vi "Add Copied Standalone VIs to Library.vi"(0 "project reference in":refnum<vi>, 5 "copied standalone VIs":cluster{"Lib path":path, "VI path":path}[](array[cluster]), 11 "error in":errorcluster) -> (4 "project reference out":refnum<vi>, 15 "error out":errorcluster)   [LabVIEW 2021, in "Multiple Converter.lvlib"]
uses:
  Multiple Converter.lvlib
  Converter Reusables/Converter Reusables.lvlib
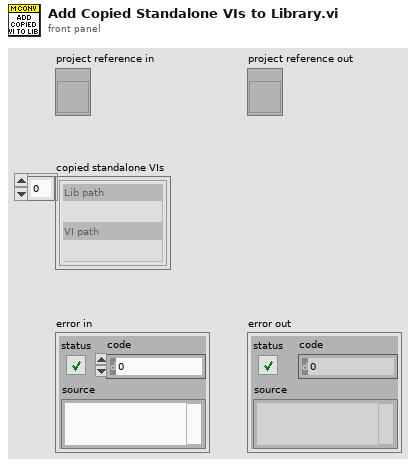
[diagram p1: front panel]
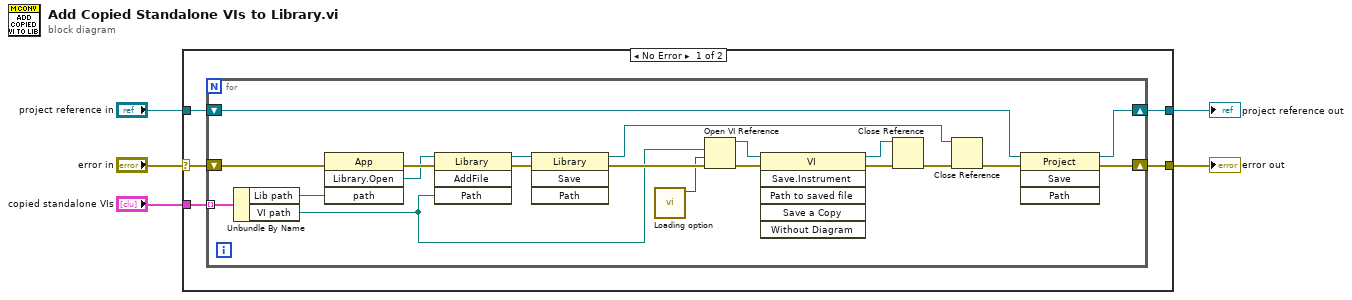
[diagram p0: block diagram]
diagram:
  n1 = case shown="No Error" "error in" {
    selector: "error in" -> [w10 w32]
    tunnel: [w9 w32] -> w4
    tunnel: "project reference in" -> [w8 w31]
    tunnel: [w7 w31] -> w2
    tunnel: "copied standalone VIs" -> [w6 _]
    frame No Error {
      n2 = for {
        shift-right: [w16] -> w9
        shift-left: w10 -> [w30]
        shift-right: [w14] -> w7
        shift-left: w8 -> [w15]
        tunnel: w6 -> [w11] mode=indexing
        n3 = Unbundle By Name(w11) -> ("Lib path"=w25:path, "VI path"=w22:path)
        n4 = invoke class="App" method="Library.Open"(error in=w30, "path"=w25) -> (error out=w29:errorcluster, "Open Library"=w24:refnum<vi>)  [unwired: 2 in, 2 out]
        n5 = invoke class="Library" method="AddFile"(reference=w24, error in=w29, "Path"=w22) -> (reference out=w26:refnum<vi>, error out=w28:errorcluster)  [unwired: 1 in, 2 out]
        n6 = invoke class="Library" method="Save"(reference=w26, error in=w28) -> (reference out=w12:refnum<vi>, error out=w27:errorcluster)  [unwired: 2 in, 2 out]
        n7 = call "Loading option.vi"() -> ("options"=w21:i32)  [unwired: 11 in]
        n8 = Open VI Reference(vi path=w22, options=w21, error in (no error)=w27) -> (vi reference=w19:refnum<vi>, error out=w23:errorcluster)  [unwired: 3 in]
        n9 = invoke class="VI" method="Save.Instrument"(reference=w19, error in=w23) -> (reference out=w17:refnum<vi>, error out=w20:errorcluster)  [unwired: 4 in, 4 out]
        n10 = Close Reference(reference=w17, error in (no error)=w20) -> (error out=w18:errorcluster)
        n11 = Close Reference(reference=w12, error in (no error)=w18) -> (error out=w13:errorcluster)
        n12 = invoke class="Project" method="Save"(reference=w15, error in=w13) -> (reference out=w14:refnum<vi>, error out=w16:errorcluster)  [unwired: 2 in, 2 out]
      }
    }
    frame Error {
    }
  }
  "error out" <- w4
  "project reference out" <- w2
